vi "Plot load reader V2.vi"(7 "First call? (init)":bool, 8 "error in (no error)":errorcluster, 9 "Load options (All)":T1={"Load plots?"=TRUE, "Load X-axis?"=TRUE, "Load Y-axes?"=TRUE, "Load General?"=TRUE}, 10 "Plot config":T2={"plots"=[], "X-axis"={"Name Label.Text"="", "Style"=0, "Tick Colors:Minor Tick Color"=0, "Tick Colors:Tick Color"=0, "Marker Colors:Text Color"=0, "Grid Colors:Major Color"=0, "Grid Colors:Minor Color"=0, "Mapping Mode"=0, "Flipped"=FALSE, "Name Label.Visible"=FALSE, "Name Label.Text Colors:Text Color"=0, "Scale Fit"=0, "Range:Maximum"=0.0, "Range:Minimum"=0.0, "Offset and Multiplier:Multiplier"=0.0, "Offset and Multiplier:Offset"=0.0, "Name Label.Font:Size"=0, "Marker.Font:Size"=0, "Uniform Marker Spacing?"=TRUE, "Format String"=""}, "Y-axes"=[], "General"={"Title"="", "Time to Plot"=1800.0, "Title.Visible"=FALSE, "Sidebar.Visible"=FALSE, "Plot Area:Colors:BG Color"=0, "X Scale.Plot Name"="", "X Scale.Use Plot Name"=FALSE}} {"General"."Time to Plot" format="%<%M:%S>t"}, 11 "Refs":T7) -> (0 "error out":errorcluster)   [LabVIEW 2021, in "RocketPlot.lvlib"]
uses:
  RocketPlot.lvlib
  TypeDefs/Plot UI references.ctl
  Classes/RocketPlotHandle/RocketPlotHandle.lvclass
  <userlib>/bjustice/TipStripOOPanel/Classes/TipPanelHandle/TipPanelHandle.lvclass
  TypeDefs/Plot top row.ctl
  TypeDefs/plot load data V2.ctl
  TypeDefs/plot properties V2.ctl
  TypeDefs/plot attributes V2.ctl
  TypeDefs/Plot scale axis properties.ctl
  TypeDefs/Plot general properties.ctl
  Classes/RocketPlotHandle/SubVIs/Load config options.ctl
  Plot default properties.vi
  Plot Load maker V2 - scalewrite wrapper.vi
  Plot attributes load.vi
  subscribed name change.vi
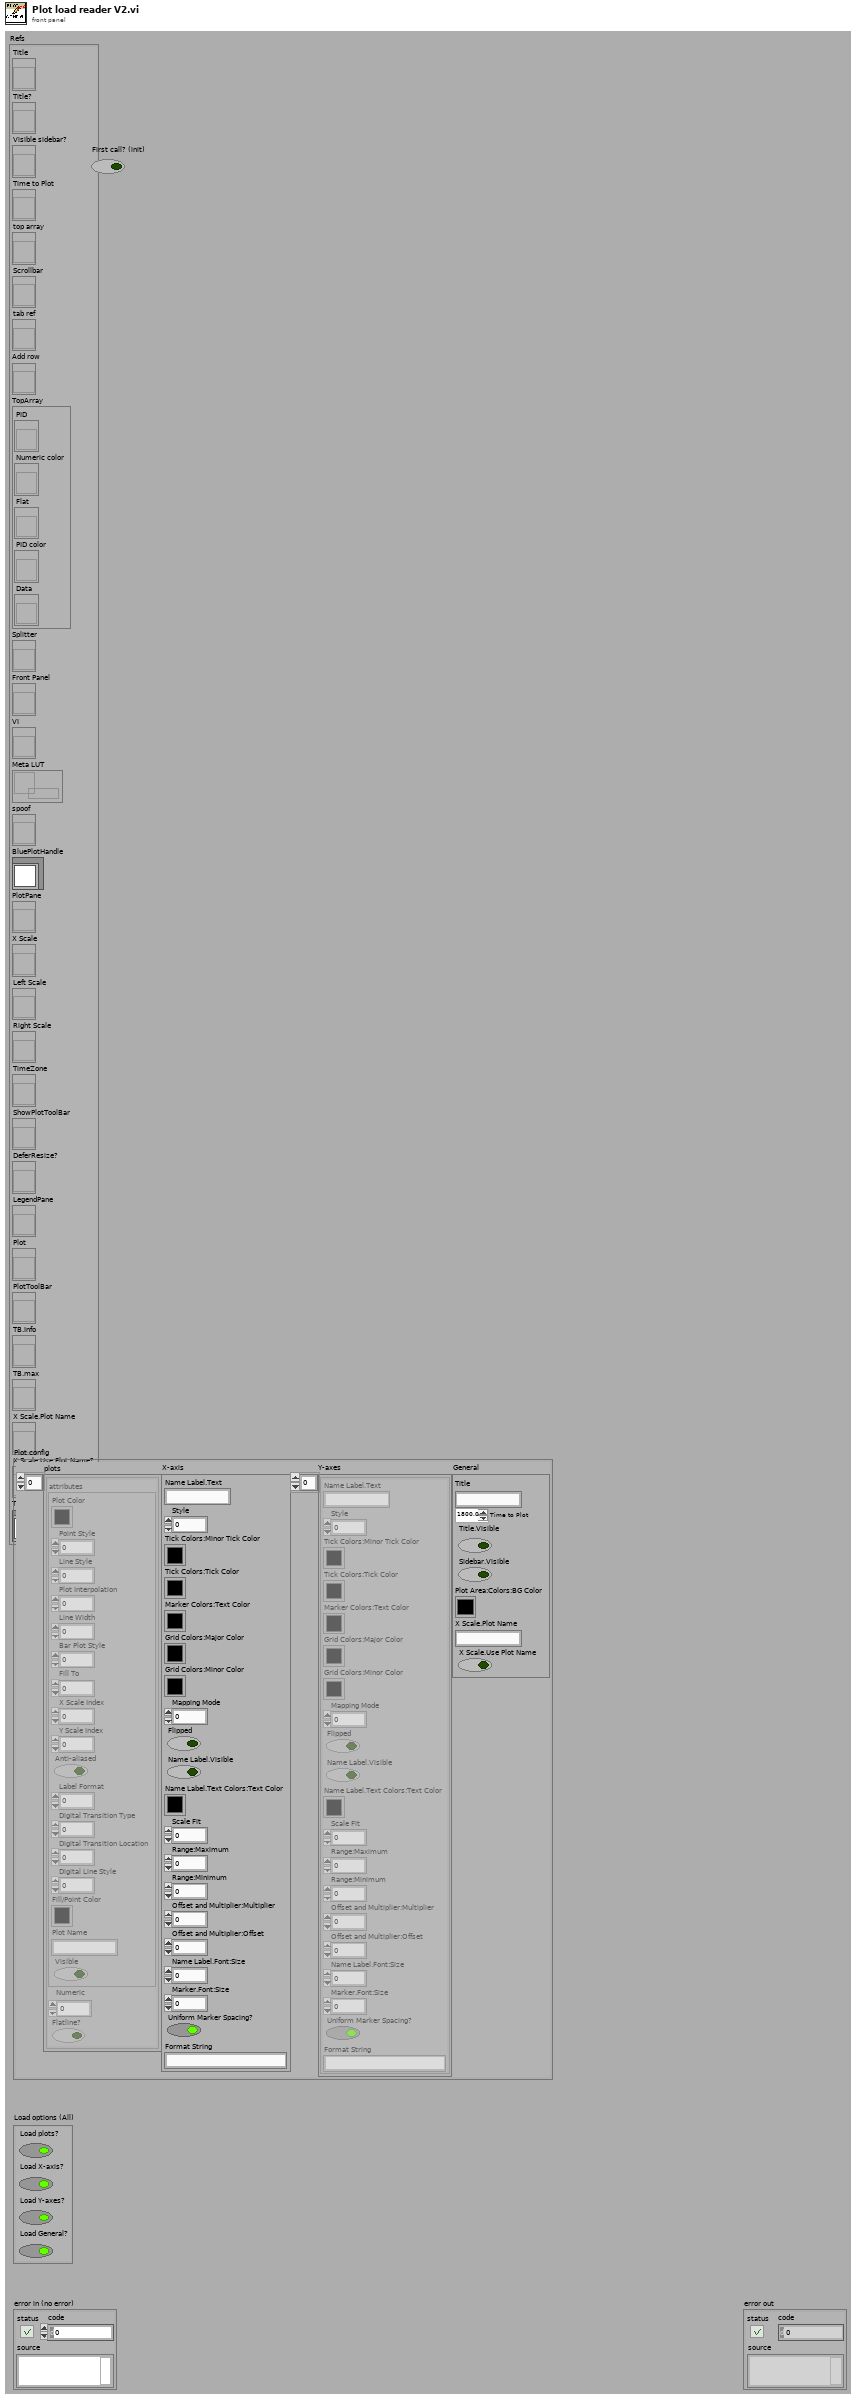
[diagram p1: front panel]
types:
  T1 = typedef "RocketPlotHandle.lvclass/Load config options.ctl" = cluster{"Load plots?":bool, "Load X-axis?":bool, "Load Y-axes?":bool, "Load General?":bool}
  T2 = typedef "RocketPlot.lvlib/plot load data V2.ctl" = cluster{"plots":T3[], "X-axis":T5, "Y-axes":T5[], "General":T6}
  T3 = typedef "RocketPlot.lvlib/plot properties V2.ctl" = cluster{"attributes":T4, "Numeric":dbl, "Flatline?":bool}
  T4 = typedef "RocketPlot.lvlib/plot attributes V2.ctl" = cluster{"Plot Color":u32, "Point Style":u8, "Line Style":u8, "Plot Interpolation":u8, "Line Width":u8, "Bar Plot Style":u8, "Fill To":i16, "X Scale Index":u32, "Y Scale Index":u32, "Anti-aliased":bool, "Label Format":u8, "Digital Transition Type":u8, "Digital Transition Location":u8, "Digital Line Style":u8, "Fill/Point Color":u32, "Plot Name":string, "Visible":bool}
  T5 = typedef "RocketPlot.lvlib/Plot scale axis properties.ctl" = cluster{"Name Label.Text":string, "Style":u8, "Tick Colors:Minor Tick Color":u32, "Tick Colors:Tick Color":u32, "Marker Colors:Text Color":u32, "Grid Colors:Major Color":u32, "Grid Colors:Minor Color":u32, "Mapping Mode":u8, "Flipped":bool, "Name Label.Visible":bool, "Name Label.Text Colors:Text Color":u32, "Scale Fit":u8, "Range:Maximum":dbl, "Range:Minimum":dbl, "Offset and Multiplier:Multiplier":dbl, "Offset and Multiplier:Offset":dbl, "Name Label.Font:Size":u32, "Marker.Font:Size":u32, "Uniform Marker Spacing?":bool, "Format String":string}
  T6 = typedef "RocketPlot.lvlib/Plot general properties.ctl" = cluster{"Title":string, "Time to Plot":dbl, "Title.Visible":bool, "Sidebar.Visible":bool, "Plot Area:Colors:BG Color":u32, "X Scale.Plot Name":string, "X Scale.Use Plot Name":bool}
  T7 = typedef "RocketPlot.lvlib/Plot UI references.ctl" = cluster{"Title":refnum<vi>, "Title?":refnum<vi>, "Visible sidebar?":refnum<vi>, "Time to Plot":refnum<vi>, "top array":refnum<vi>, "Scrollbar":refnum<vi>, "tab ref":refnum<vi>, "Add row":refnum<vi>, "TopArray":cluster{"PID":refnum<vi>, "Numeric color":refnum<vi>, "Flat":refnum<vi>, "PID color":refnum<vi>, "Data":refnum<vi>}, "Splitter":refnum<vi>, "Front Panel":refnum<vi>, "VI":refnum<vi>, "Meta LUT":refnum<data-value>, "spoof":refnum<vi>, "BluePlotHandle":refnum<class "RocketPlotHandle.lvclass">, "PlotPane":refnum<vi>, "X Scale":refnum<vi>, "Left Scale":refnum<vi>, "Right Scale":refnum<vi>, "TimeZone":refnum<vi>, "ShowPlotToolBar":refnum<vi>, "DeferResize?":refnum<vi>, "LegendPane":refnum<vi>, "Plot":refnum<vi>, "PlotToolBar":refnum<vi>, "TB.Info":refnum<vi>, "TB.max":refnum<vi>, "X Scale.Plot Name":refnum<vi>, "X Scale.Use Plot Name?":refnum<vi>, "TipPanel":refnum<class "TipPanelHandle.lvclass">}
  T8 = typedef "Plot top row.ctl" = cluster{"PID":string, "index":i32, "PID color":u32, "right axis?":bool, "Flatline?":bool, "Numeric color":u32, "Data":string, "Flat":string}
  T9 = typedef "RocketPlot.lvlib/Plot top row.ctl" = cluster{"PID":string, "index":i32, "PID color":u32, "right axis?":bool, "Flatline?":bool, "Numeric color":u32, "Data":string, "Flat":string}
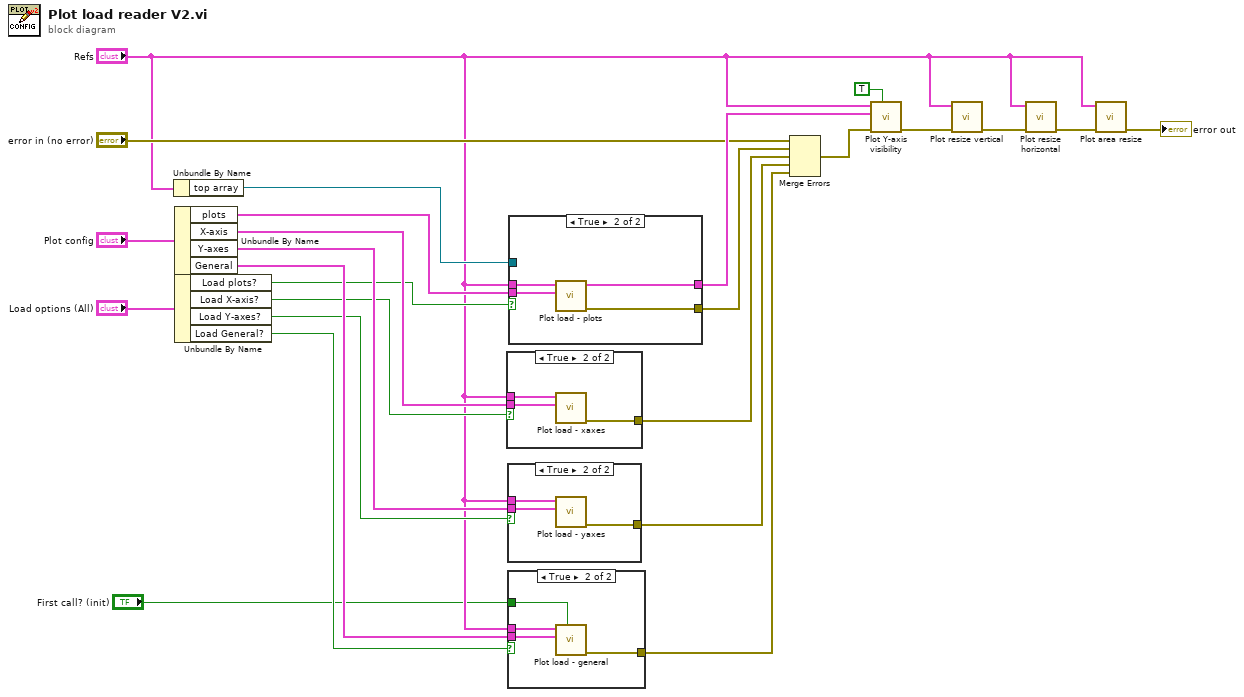
[diagram p0: block diagram]
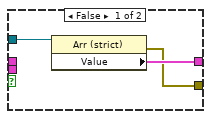
[diagram p2: hidden frame]
diagram:
  n1 = Unbundle By Name("Refs") -> ("top array"=w14:refnum<vi>)
  n2 = Unbundle By Name("Plot config") -> ("plots"=w16:T3[], "X-axis"=w18:T5, "Y-axes"=w20:T5[], "General"=w21:T6)
  n3 = Unbundle By Name("Load options (All)") -> ("Load plots?"=w11:bool, "Load X-axis?"=w10:bool, "Load Y-axes?"=w9:bool, "Load General?"=w8:bool)
  n4 = case shown="True" w10 {
    tunnel: w18 -> [_ w28]
    tunnel: [_ w27] -> w17
    tunnel: "Refs" -> [_ w26]
    frame False {
    }
    frame True {
      n5 = call "Plot load - xaxes.vi"("X-axis"=w28, "Refs"=w26) -> ("error out"=w27:errorcluster)  [unwired: 9 in]
    }
  }
  n6 = case shown="True" w9 {
    tunnel: w20 -> [_ w31]
    tunnel: [_ w30] -> w19
    tunnel: "Refs" -> [_ w29]
    frame False {
    }
    frame True {
      n7 = call "Plot load - yaxes.vi"("Y-axes"=w31, "Refs"=w29) -> ("error out"=w30:errorcluster)  [unwired: 9 in]
    }
  }
  n8 = case shown="True" w8 {
    tunnel: [_ w35] -> w6
    tunnel: w21 -> [_ w34]
    tunnel: "First call? (init)" -> [_ w33]
    tunnel: "Refs" -> [_ w32]
    frame False {
    }
    frame True {
      n9 = call "Plot load - general.vi"("First call? (init)"=w33, "General"=w34, "Refs"=w32) -> ("error out"=w35:errorcluster)  [unwired: 8 in]
    }
  }
  n10 = case shown="True" w11 {
    tunnel: w16 -> [_ w42]
    tunnel: [w38 w41] -> w7
    tunnel: "Refs" -> [_ w40]
    tunnel: [w36 w39] -> w15
    tunnel: w14 -> [w37 _]
    frame False {
      n11 = property class="Arr (strict)"(reference=w37) -> (error out=w36:errorcluster, "Value"=w38:T8[])  [unwired: 1 in, 1 out]
    }
    frame True {
      n12 = call "Plot load - plots.vi"("plots"=w42, "Refs"=w40) -> ("error out"=w39:errorcluster, "top array.value"=w41:T9[])  [unwired: 8 in]
    }
  }
  n13 = Merge Errors("error in (no error)", w15, w17, w19, w6) -> (w2:errorcluster)
  n14 = call "Plot Y-axis visibility.vi"("Force update? (F)"=TRUE, "error in (no error)"=w2, "top array"=w7, "Refs"="Refs") -> ("error out"=w4:errorcluster)  [unwired: 7 in]
  n15 = call "Plot resize vertical.vi"("error in (no error)"=w4, "Refs"="Refs") -> ("error out"=w25:errorcluster)  [unwired: 7 in, 2 out]
  n16 = call "Plot resize horizontal.vi"("error in (no error)"=w25, "Refs"="Refs") -> ("error out"=w23:errorcluster)  [unwired: 9 in]
  n17 = call "Plot area resize.vi"("error in (no error)"=w23, "Refs"="Refs") -> ("error out"=→"error out":errorcluster)  [unwired: 9 in]
